vi "ParseIPControl.vi"(0 "data out":string, 1 "offset":u8) -> (2 "Bytes Read":i32, 3 "srcId":u8, 4 "data":i16)   [LabVIEW 2009]
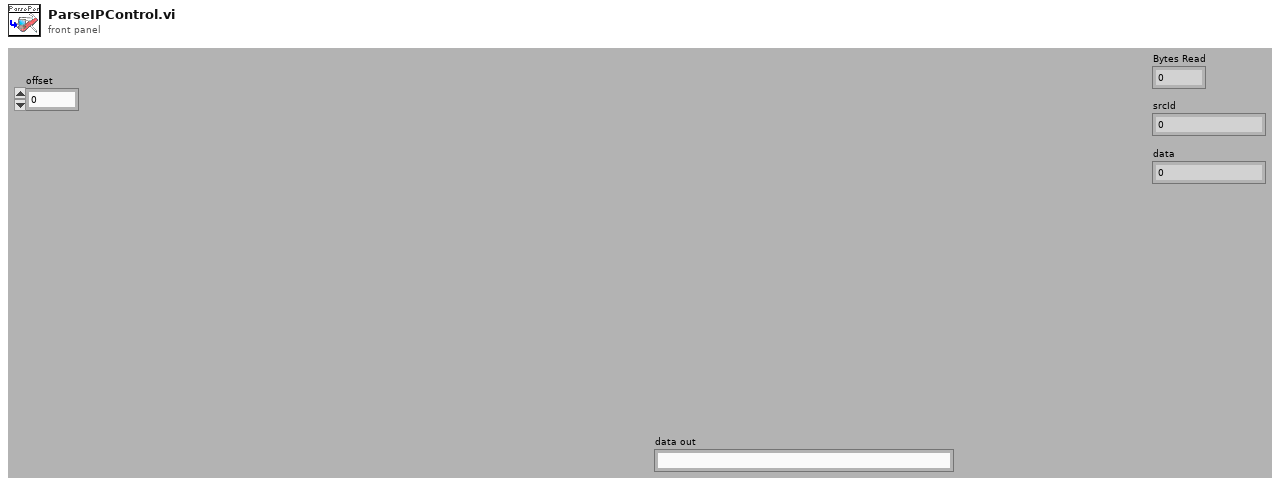
[diagram p1: front panel]
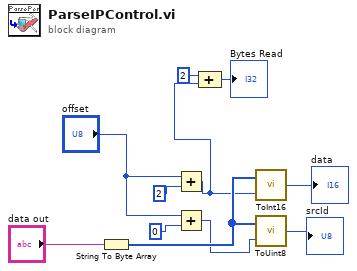
[diagram p0: block diagram]
diagram:
  n1 = String To Byte Array(string="data out") -> (unsigned byte array=w10:u8[])
  n2 = Add(x="offset", y=2 ("index")) -> (x+y=w1:i32)
  n3 = Add(x="offset", y=0 ("index")) -> (x+y=w4:i32)
  n4 = Compound Arithmetic op=ADD(2 ("value"), w1) -> (→"Bytes Read":i32)
  n5 = call "ToInt16.vi"("index"=w1, "array"=w10) -> ("sp float"=→"data":i16)
  n6 = call "ToUint8.vi"("index"=w4, "array"=w10) -> ("sp float"=→"srcId":u8)
